vi "Design a Fixed-Point Highpass Filter.vi"() -> ()   [LabVIEW 2023]
uses:
  <vilib>/addons/Digital Filter Design/FXPModel.llb/DFD FXP Quantize Coef (Easy).vi
  <vilib>/Utility/VariantDataType/GetNumericFxpInfo.vi
  <vilib>/addons/Digital Filter Design/FXPSim.llb/dfd_Check Input FXP Settings.vi
  <vilib>/addons/Digital Filter Design/FXPSim.llb/dfd_Check SRate Simulation Integer Input.vi
  <vilib>/addons/Digital Filter Design/FXPSim.llb/dfd_FXP Simu.vi
  <vilib>/addons/Digital Filter Design/FilterLib.llb/DFD Save Filter to File.vi
  <vilib>/addons/Digital Filter Design/_Objects.llb/DFD Quantization Sources.ctl
  <vilib>/addons/Digital Filter Design/_Objects.llb/DFD FXP Statistics Data.ctl
  <vilib>/addons/Digital Filter Design/FXPSim.llb/SimXnode/DFD FXP Simulation.xnode
  <vilib>/addons/Digital Filter Design/_Objects.llb/DFD Filter Obj.ctl
  <vilib>/addons/Digital Filter Design/_Objects.llb/DFD Filter Coef.ctl
  <vilib>/addons/Digital Filter Design/_Objects.llb/DFD Filter Structure Type Selector.ctl
  <vilib>/addons/Digital Filter Design/_Objects.llb/dfd_Internal Quantization Settings.ctl
  <vilib>/addons/Digital Filter Design/_Objects.llb/dfd_Internal Quantization Srcs.ctl
  <vilib>/addons/Digital Filter Design/_Objects.llb/DFD Coef Norm Type.ctl
  <vilib>/addons/Digital Filter Design/NI_DigFilterLicensed.lvlib
  <vilib>/addons/Digital Filter Design/NI_DigFilter_FXP.lvlib
  <vilib>/Utility/VariantDataType/VariantType.lvlib
panel:
  out "Error Message":string
  in  "Save Filter to File":bool
  in  "Signal from DAQ Device":fxp<+/-,20,5>[](array[numeric])=[-0.329681396484375, -4.286834716796875, 9.429473876953125, -8.305145263671875, -0.662689208984375, -2.729522705078125, 7.085845947265625, -3.488800048828125, 2.225128173828125, 3.63323974609375, -5.179962158203125, 7.238677978515625, 4.8243408203125, 2.791412353515625, -9.072296142578125, -1.45458984375, 9.80548095703125, 7.69830322265625, -9.72210693359375, 1.994598388671875, -6.56597900390625, 5.69097900390625, 8.246246337890625, -2.866546630859375, -6.74896240234375, -7.206298828125, -4.030517578125, 6.043731689453125, 8.05010986328125, 3.516815185546875, 9.917205810546875, -8.699188232421875, 0.4688720703125, 0.513763427734375, 4.93695068359375, 5.129974365234375, -7.52783203125, 7.8001708984375, 1.576171875, 2.575714111328125, -4.20550537109375, -1.79620361328125, -5.672332763671875, 7.192901611328125, 9.375030517578125, -2.6258544921875, -5.70220947265625, 4.27691650390625, -0.683868408203125, 4.7548828125, 7.179962158203125, 7.098846435546875, -4.2564697265625, -8.908050537109375, -3.31884765625, 5.65350341796875, 0.428924560546875, 1.617706298828125, 7.4306640625, 4.920562744140625, -7.7008056640625, -7.17559814453125, -4.438934326171875, 8.03948974609375, 6.6856689453125, -2.220062255859375, -5.266357421875, -9.69549560546875, -7.25823974609375, 3.82177734375, 6.288909912109375, -1.042572021484375, 1.600128173828125, 8.114593505859375, 3.807037353515625, 7.95660400390625, -4.94366455078125, 0.53521728515625, 5.354522705078125, 5.111419677734375, 5.87420654296875, 5.844146728515625, 7.76446533203125, 6.58843994140625, 2.994964599609375, 0.97381591796875, 4.075286865234375, -2.38446044921875, -8.872802734375, 7.240264892578125, 3.440216064453125, -3.22064208984375, 7.457244873046875, -8.672027587890625, -7.299957275390625, -7.650421142578125, -8.7384033203125, -2.68670654296875, -0.992645263671875, 7.793701171875, -7.697601318359375, -1.930633544921875, 7.630767822265625, 8.330291748046875, -8.08685302734375, -8.128021240234375, 2.206024169921875, -2.2911376953125, -7.6170654296875, -6.148284912109375, -9.52166748046875, -5.676300048828125, 9.081939697265625, -1.682403564453125, -0.28973388671875, 2.24139404296875, -2.659698486328125, -9.855255126953125, 1.220489501953125, 2.930938720703125, 9.869171142578125, -2.096160888671875, 4.275848388671875, 0.7493896484375, 7.155364990234375, 8.169921875, 2.828765869140625, 8.2470703125] format="%.6g"
  out "Filtered Signals":dbl[](graph)
  # "Design a fixed-point highpass filter"
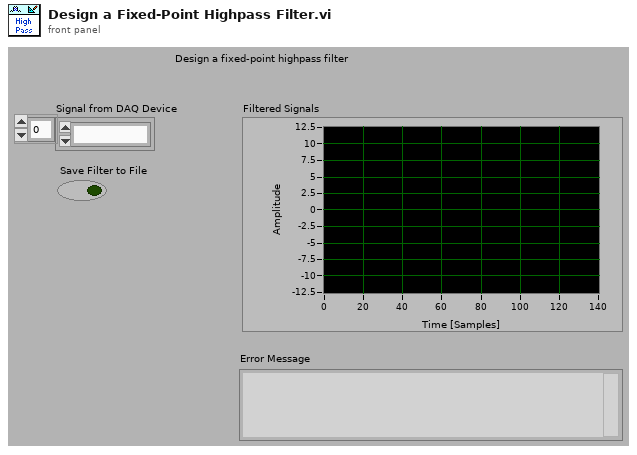
[diagram p1: front panel]
types:
  T1 = typedef "NI_DigFilterLicensed.lvlib/DFD Filter Obj.ctl" = cluster{"mSRate_Fs":dbl, "mSRate_Version":string, "mSRate_Comments":string, "mSRate_OrgCoef":T2, "mSRate_CurCoef":T2, "mSRate_Quantized?":bool, "mSRate_QCoef":T2, "mSRate_QSettings":T4[], "mSRate_Order":i32, "mSRate_Scaling":cluster{"mSRate_ScaleByPowerOf2?":bool, "mSRate_ScaleType":T6}}
  T2 = typedef "NI_DigFilterLicensed.lvlib/DFD Filter Coef.ctl" = cluster{"type":T3, "gain":dbl, "coef a (k)":dbl[], "coef b (v)":dbl[]}
  T3 = typedef "NI_DigFilterLicensed.lvlib/DFD Filter Structure Type Selector.ctl" = enum16{"Undefined", "FIR Direct Form", "FIR Direct Form Transposed", "FIR Symmetric", "FIR Antisymmetric", "IIR Direct Form I", "IIR Direct Form I Transposed", "IIR Direct Form II", "IIR Direct Form II Transposed", "IIR Cascaded Second Order Sections Form I", "IIR Cascaded Second Order Sections Form I Transposed", "IIR Cascaded Second Order Sections Form II", "IIR Cascaded Second Order Sections Form II Transposed", "Lattice Allpass (basic sections)", "Lattice Allpass (one multiplier sections)", "Lattice Allpass (normalized sections)", "Lattice AR (basic sections)", "Lattice AR (one multiplier sections)", "Lattice AR (normalized sections)", "Lattice MA (minimum phase)", "Lattice MA (maximum phase)", "Lattice ARMA (basic sections)", "Lattice ARMA (one multiplier sections)", "Lattice ARMA (normalized sections)"}
  T4 = typedef "NI_DigFilterLicensed.lvlib/dfd_Internal Quantization Settings.ctl" = cluster{"source":T5, "wl":i16, "iwl":i16, "overflow mode":enum16{"Saturation", "Wrap"}, "rounding mode":enum16{"Nearest", "Truncation"}, "signed?":bool}
  T5 = typedef "NI_DigFilterLicensed.lvlib/dfd_Internal Quantization Srcs.ctl" = u16
  T6 = typedef "NI_DigFilterLicensed.lvlib/DFD Coef Norm Type.ctl" = enum16{"No Norm", "Time Domain 1-Norm", "Time Domain 2-Norm", "Time Domain Inf-Norm"}
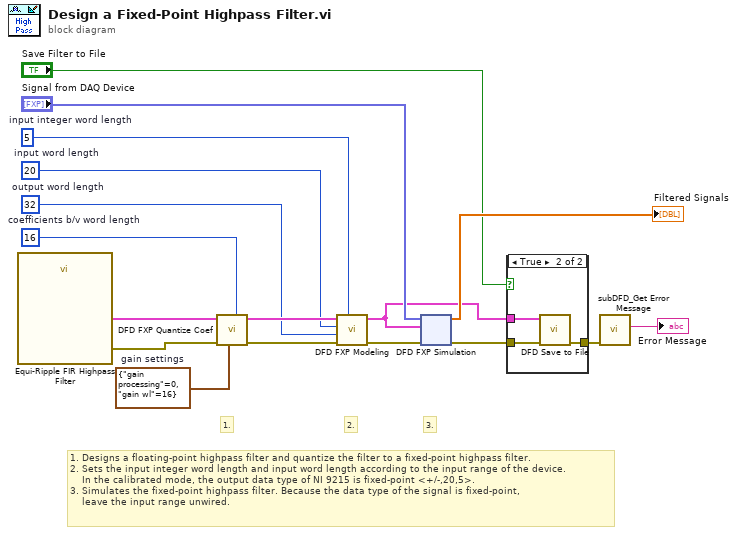
[diagram p0: block diagram]
diagram:
  w10 = i16 5  # input integer word length
  w11 = i16 32  # output word length
  w12 = i16 20  # input word length
  w15 = i16 16  # coefficients b/v word length
  w14 = cluster{"gain processing":u16, "gain wl":i16} {"gain processing"=0, "gain wl"=16}  # gain settings
  # "1."
  # "3."
  # "2."
  # "1. Designs a floating-point highpass filter and quantize the filter to a fixed-point highpass filter.\n2. Sets the input integer word length and input word length according to the input range of the device. \n    In the calibrated mode, the output data type of NI 9215 is fixed-point <+/-,20,5>. \n3. Simulates the fixed-point highpass filter. Because the data type of the signal is fixed-point, \n    leave the input range unwired."
  n1 = call "Equi-Ripple FIR Highpass Filter"() -> ("error out"=w2:errorcluster, "filter out"=w3:T1)  [unwired: 1 in, 9 out]
  n2 = call-poly <vilib>:"DFD FXP Quantize Coef.vi"("coefficients b/v word length"=w15, "gain settings"=w14, "error in (no error)"=w2, "filter in"=w3) -> ("error out"=w16:errorcluster, "filter out"=w17:T1)  [unwired: 1 in, 5 out]
  n3 = call <vilib>:"DFD FXP Modeling.vi"("input integer word length"=w10, "error in (no error)"=w16, "output word length"=w11, "input word length"=w12, "filter in"=w17) -> ("error out"=w13:errorcluster, "filter out"=w6:T1)  [unwired: 2 in, 3 out]
  n4 = xnode "DFD FXP Simulation"("error in (no error)"=w13, "filter in"=w6, "signal in"="Signal from DAQ Device") -> ("error out"=w7:errorcluster, "DBL signal out"=→"Filtered Signals":dbl[])  [unwired: 2 in, 3 out]
  n5 = case shown="True" "Save Filter to File" {
    tunnel: w7 -> [w18 w21]
    tunnel: w6 -> [_ w20]
    tunnel: [w18 w19] -> w4
    frame False {
    }
    frame True {
      n6 = call-poly <vilib>:"DFD Save to File.vi"("error in (no error)"=w21, "filter in"=w20) -> ("error out"=w19:errorcluster)  [unwired: 2 in, 7 out]
    }
  }
  n7 = call <vilib>:"subDFD_Get Error Message.vi"("error in (no error)"=w4) -> ("Error Message"=→"Error Message":string)  [unwired: 10 out]
